vi "UDP Data Link - Configuration Utilities - Get System Mappings.vi"(8 "error in (no error)":errorcluster, 11 "Item Ref in":T1 format="%.0x") -> (0 "error out":errorcluster, 1 "Channel Path Destinations":string[](array[string]), 2 "Channel Path Sources":string[](array[string]), 3 "Item Ref out":T1 format="%.0x")   [LabVIEW 2015, in "UDP-Custom-Device System Explorer.lvlib"]
uses:
  UDP-Custom-Device System Explorer.lvlib
  <vilib>/NI Veristand/Custom Device API/Custom Device Item Ref.ctl
  NationalInstruments.VeriStand.SystemDefinitionAPI
  <vilib>/NI VeriStand/Custom Device API/Custom Device API.lvlib
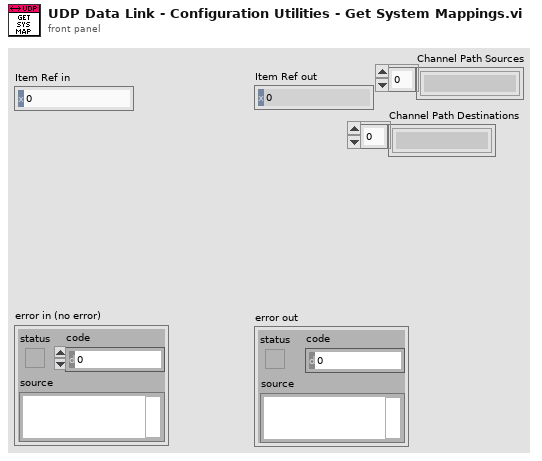
[diagram p1: front panel]
types:
  T1 = typedef "Custom Device API.lvlib/Custom Device Item Ref.ctl" = u64
  T2 = typedef "Custom Device API.lvlib/Custom Device Pointer.ctl" = refnum<k24>
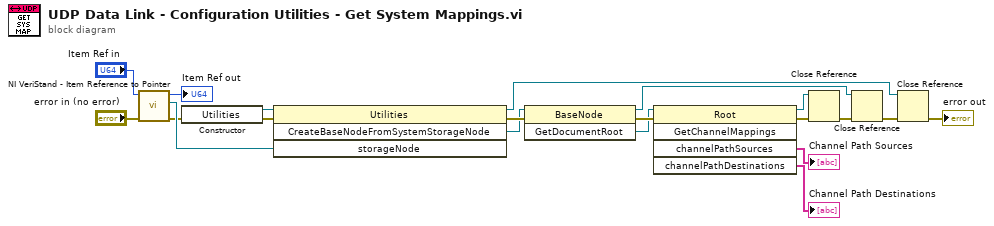
[diagram p0: block diagram]
diagram:
  n1 = call <vilib>:"NI VeriStand - Item Reference to Pointer.vi"("error in (no error)"="error in (no error)", "Item Ref in"="Item Ref in") -> ("error out"=w2:errorcluster, "Node Pointer"=w8:T2, "Item Ref out"=→"Item Ref out":T1)  [unwired: 6 in, 1 out]
  n2 = constructor class="Utilities"(error in=w2) -> (reference out=w9:refnum<k24>, error out=w1:errorcluster)  [unwired: 2 in, 1 out]
  n3 = invoke class="Utilities" method="CreateBaseNodeFromSystemStorageNode"(reference=w9, error in=w1, "storageNode"=w8) -> (reference out=w19:refnum<k24>, error out=w12:errorcluster, "CreateBaseNodeFromSystemStorageNode"=w10:refnum<k24>)  [unwired: 1 in, 1 out]
  n4 = invoke class="BaseNode" method="GetDocumentRoot"(reference=w10, error in=w12) -> (reference out=w17:refnum<k24>, error out=w13:errorcluster, "GetDocumentRoot"=w11:refnum<k24>)  [unwired: 1 in]
  n5 = invoke class="Root" method="GetChannelMappings"(reference=w11, error in=w13) -> (reference out=w15:refnum<k24>, error out=w14:errorcluster, "channelPathSources"=→"Channel Path Sources":string[], "channelPathDestinations"=→"Channel Path Destinations":string[])  [unwired: 3 in, 1 out]
  n6 = Close Reference(reference=w15, error in (no error)=w14) -> (error out=w16:errorcluster)
  n7 = Close Reference(reference=w17, error in (no error)=w16) -> (error out=w18:errorcluster)
  n8 = Close Reference(reference=w19, error in (no error)=w18) -> (error out=→"error out":errorcluster)
